vi "Post-Install Custom Action.vi"(10 "Variant":variant) -> (0 "error out":errorcluster)   [LabVIEW 2020]
panel:
  out "Path":path
  out "Numeric":i32
  out "size(s) 2":i32
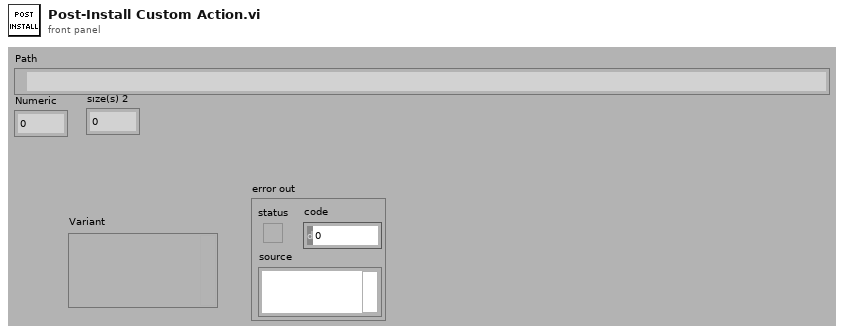
[diagram p1: front panel]
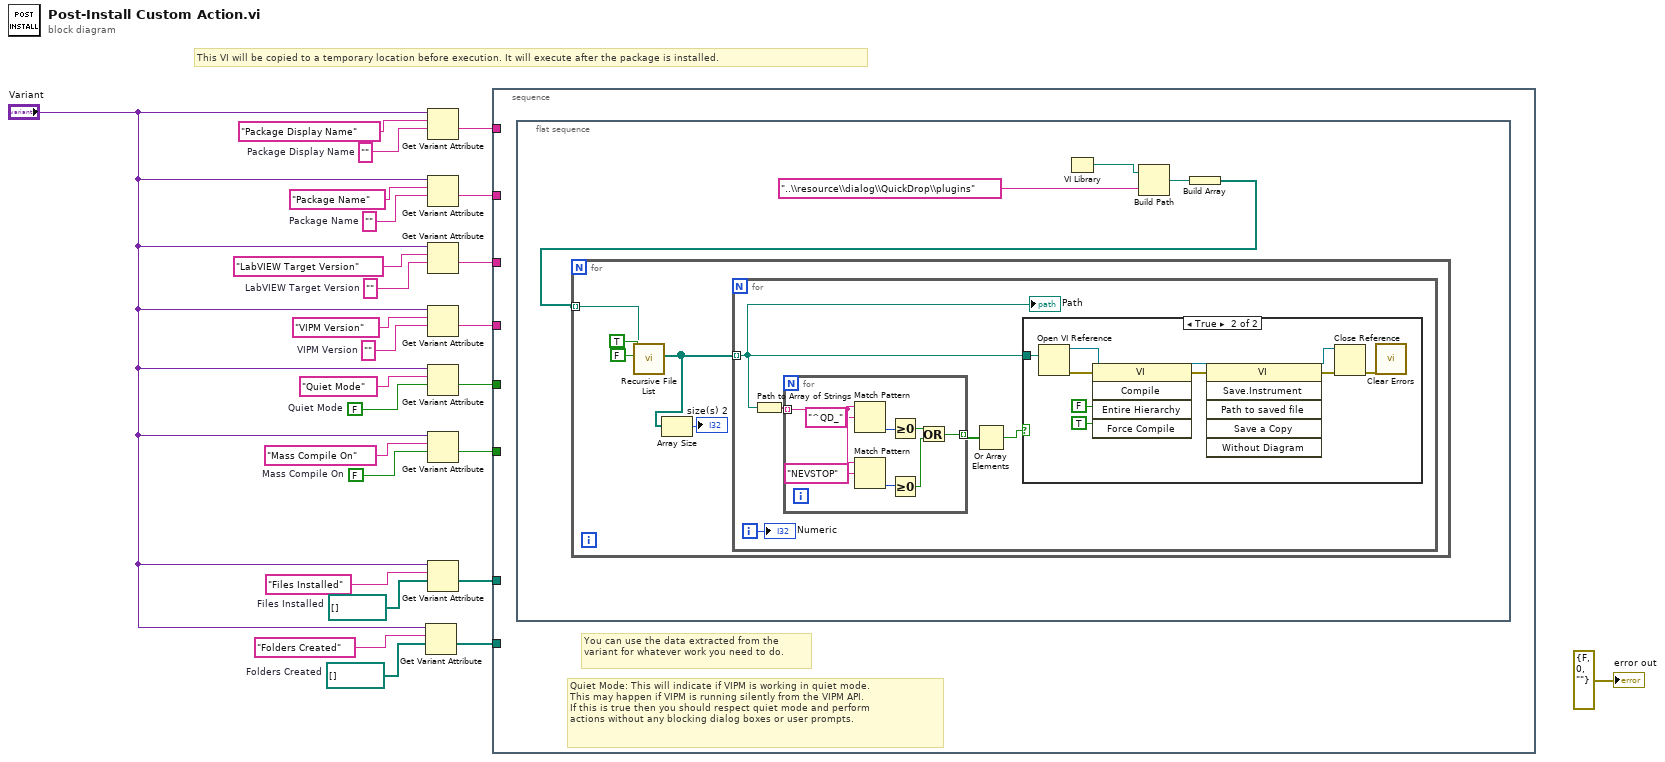
[diagram p0: block diagram]
diagram:
  w1 = path[] []  # Folders Created
  w2 = path[] []  # Files Installed
  w8 = FALSE  # Mass Compile On
  w9 = ""  # Package Display Name
  w16 = FALSE  # Quiet Mode
  w19 = ""  # VIPM Version
  w21 = ""  # LabVIEW Target Version
  w23 = ""  # Package Name
  # "This VI will be copied to a temporary location before execution. It will execute after the package is installed."
  n1 = Get Variant Attribute(Variant="Variant", name="Folders Created", default value (empty Variant)=w1) -> (value=w6:path[])  [unwired: 1 in, 3 out]
  n2 = Get Variant Attribute(Variant="Variant", name="Package Display Name", default value (empty Variant)=w9) -> (value=w15:string)  [unwired: 1 in, 3 out]
  n3 = Get Variant Attribute(Variant="Variant", name="Package Name", default value (empty Variant)=w23) -> (value=w14:string)  [unwired: 1 in, 3 out]
  n4 = Get Variant Attribute(Variant="Variant", name="LabVIEW Target Version", default value (empty Variant)=w21) -> (value=w13:string)  [unwired: 1 in, 3 out]
  n5 = Get Variant Attribute(Variant="Variant", name="VIPM Version", default value (empty Variant)=w19) -> (value=w12:string)  [unwired: 1 in, 3 out]
  n6 = Get Variant Attribute(Variant="Variant", name="Quiet Mode", default value (empty Variant)=w16) -> (value=w11:bool)  [unwired: 1 in, 3 out]
  n7 = Get Variant Attribute(Variant="Variant", name="Mass Compile On", default value (empty Variant)=w8) -> (value=w10:bool)  [unwired: 1 in, 3 out]
  n8 = Get Variant Attribute(Variant="Variant", name="Files Installed", default value (empty Variant)=w2) -> (value=w5:path[])  [unwired: 1 in, 3 out]
  n9 = stacked-sequence {
    tunnel: w15 -> [_]
    tunnel: w14 -> [_]
    tunnel: w13 -> [_]
    tunnel: w12 -> [_]
    tunnel: w11 -> [_]
    tunnel: w10 -> [_]
    tunnel: w5 -> [_]
    tunnel: w6 -> [_]
    frame #0 {
      # "Quiet Mode: This will indicate if VIPM is working in quiet mode.\nThis may happen if VIPM is running silently from the VIPM API.\nIf this is true then you should respect quiet mode and perform\nactions without any blocking dialog boxes or user prompts."
      # "You can use the data extracted from the variant for whatever work you need to do."
      n10 = flat-sequence {
        frame #0 {
          n11 = VI Library() -> (path=w29:path)
          n12 = Build Path(base path=w29, name or relative path="..\\resource\\dialog\\QuickDrop\\plugins") -> (appended path=w30:path)
          n13 = Build Array(w30) -> (w27:path[])
          n14 = for {
            tunnel: w27 -> [w33] mode=indexing
            n15 = call <vilib>:"Recursive File List.vi"("Continue Recursing on Error? (F)"=TRUE, "Treat LLBs as Folders?"=FALSE, "Folder Path"=w33) -> ("All Files in Dir"=w32:path[])  [unwired: 4 in, 4 out]
            n16 = Array Size(array=w32) -> (size(s)=→"size(s) 2":i32)
            n17 = for {
              tunnel: w32 -> [w39] mode=indexing
              i -> [w40]
              n18 = Path to Array of Strings(0:w39) -> (2:w38:string[])  [unwired: 1 out]
              n19 = for {
                tunnel: w38 -> [w48] mode=indexing
                tunnel: [w41] -> w37 mode=indexing
                n20 = Match Pattern(string=w48, regular expression="^QD_") -> (offset past match=w45:i32)  [unwired: 1 in, 3 out]
                n21 = Match Pattern(string=w48, regular expression="NEVSTOP") -> (offset past match=w44:i32)  [unwired: 1 in, 3 out]
                n22 = Greater Or Equal To 0?(x=w45) -> (x >= 0?=w43:bool)
                n23 = Greater Or Equal To 0?(x=w44) -> (x >= 0?=w42:bool)
                n24 = Or(x=w43, y=w42) -> (x .or. y?=w41:bool)
              }
              n25 = Or Array Elements(Boolean array=w37) -> (logical OR=w36:bool)
              n26 = case shown="True" w36 {
                tunnel: w39 -> [_ w56]
                frame False {
                }
                frame True {
                  n27 = Open VI Reference(vi path=w56) -> (vi reference=w54:refnum<vi>, error out=w55:errorcluster)  [unwired: 5 in]
                  n28 = invoke class="VI" method="Compile"(reference=w54, error in=w55, "Entire Hierarchy"=FALSE ("Compile Entire Hierarchy (F)"), "Force Compile"=TRUE ("Force Compile (T)")) -> (reference out=w53:refnum<vi>, error out=w52:errorcluster)  [unwired: 1 in, 3 out]
                  n29 = invoke class="VI" method="Save.Instrument"(reference=w53, error in=w52) -> (reference out=w50:refnum<vi>, error out=w51:errorcluster)  [unwired: 4 in, 4 out]
                  n30 = Close Reference(reference=w50, error in (no error)=w51) -> (error out=w49:errorcluster)
                  n31 = call <vilib>:"Clear Errors.vi"("error in (no error)"=w49) -> ()  [unwired: 5 in, 2 out]
                }
              }
              "Path" <- w39
              "Numeric" <- w40
            }
          }
        }
      }
    }
  }
  "error out" <- errorcluster {"status"=FALSE, "code"=0, "source"=""} ("error out")
